vi "CtrlTreeUpdateModifiedState.vi"(7 "Selection":string, 10 "ControlTree in":refnum<vi>, 11 "SavedSettings in":refnum<vi>) -> (1 "Boolean":bool)   [LabVIEW 2020]
panel:
  in  "error in (no error)":errorcluster
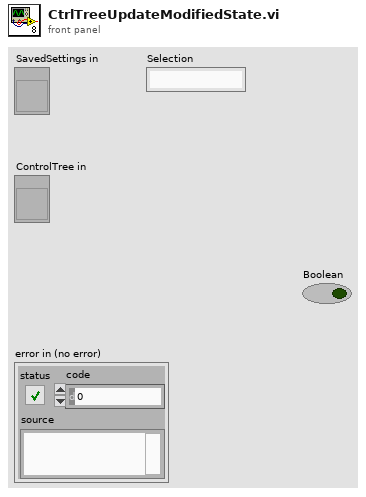
[diagram p1: front panel]
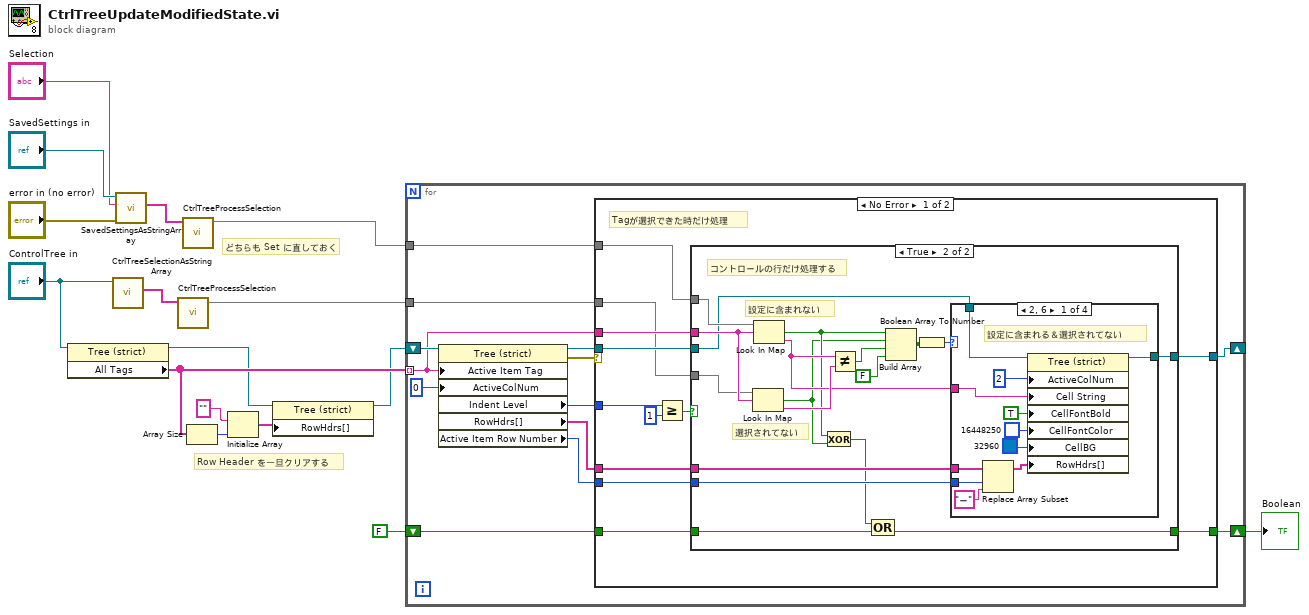
[diagram p0: block diagram]
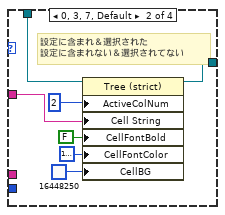
[diagram p3: hidden frame]
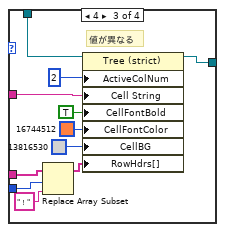
[diagram p4: hidden frame]
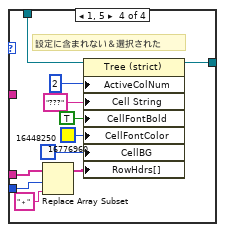
[diagram p5: hidden frame]
diagram:
  # "Row Header を一旦クリアする"
  # "どちらも Set に直しておく"
  n1 = property class="Tree (strict)"(reference="ControlTree in") -> (reference out=w6:refnum<vi>, "All Tags"=w9:string[])  [unwired: 1 in, 1 out]
  n2 = call "CtrlTreeSelectionAsStringArray.vi"("TreeControl in"="ControlTree in") -> ("Selection"=w15:string[])  [unwired: 8 in, 2 out]
  n3 = call "SavedSettingsAsStringArray.vi"("error in (no error)"="error in (no error)", "Tag"="Selection", "SavedSettings in"="SavedSettings in") -> ("Selection"=w2:string[])  [unwired: 4 in, 4 out]
  n4 = call "CtrlTreeProcessSelection.vi"("Selection"=w15) -> ("Map"=w4:map{string, string})  [unwired: 10 in]
  n5 = call "CtrlTreeProcessSelection.vi"("Selection"=w2) -> ("Map"=w3:map{string, string})  [unwired: 10 in]
  n6 = Array Size(array=w9) -> (size(s)=w10:i32)
  n7 = Initialize Array("", w10) -> (w7:string[])
  n8 = property class="Tree (strict)"(reference=w6, "RowHdrs[]"=w7) -> (reference out=w5:refnum<vi>)  [unwired: 1 in, 1 out]
  n9 = for {
    tunnel: w9 -> [w26] mode=indexing
    tunnel: w4 -> [w23]
    tunnel: w3 -> [w24]
    shift-right: [w21] -> w12
    shift-left: FALSE -> [w20]
    shift-right: [w17] -> _
    shift-left: w5 -> [w29]
    n10 = property class="Tree (strict)"(reference=w29, "Active Item Tag"=w26, "ActiveColNum"=0 ("Active Cell:Active Column Number")) -> (reference out=w27:refnum<vi>, error out=w22:errorcluster, "Indent Level"=w25:i32, "RowHdrs[]"=w19:string[], "Active Item Row Number"=w18:i32)  [unwired: 1 in]
    n11 = case shown="No Error" w22 {
      tunnel: w27 -> [w41 w102]
      tunnel: w26 -> [w40 _]
      tunnel: w25 -> [w39 _]
      tunnel: w24 -> [w38 _]
      tunnel: w23 -> [w37 _]
      tunnel: [w36 w103] -> w21
      tunnel: w20 -> [w35 w103]
      tunnel: w19 -> [w34 _]
      tunnel: w18 -> [w33 _]
      tunnel: [w32 w102] -> w17
      frame No Error {
        # "Tagが選択できた時だけ処理"
        n12 = Greater Or Equal?(x=w39, y=1) -> (x >= y?=w30:bool)
        n13 = case shown="True" w30 {
          tunnel: w40 -> [_ w60]
          tunnel: w38 -> [_ w59]
          tunnel: w37 -> [_ w58]
          tunnel: w41 -> [w42 w54]
          tunnel: [w43 w51] -> w36
          tunnel: w35 -> [w43 w52]
          tunnel: w34 -> [_ w50]
          tunnel: w33 -> [_ w49]
          tunnel: [w42 w44] -> w32
          frame False {
          }
          frame True {
            # "コントロールの行だけ処理する"
            # "設定に含まれない"
            # "選択されてない"
            n14 = Look In Map(map=w58, key=w60) -> (key not found?=w46:bool, value=w61:string)  [unwired: 1 in]
            n15 = Look In Map(map=w59, key=w60) -> (key not found?=w47:bool, value=w53:string)  [unwired: 1 in]
            n16 = Exclusive Or(1:w46, 2:w47) -> (0:w45:bool)
            n17 = Not Equal?(x=w53, y=w61) -> (x != y?=w57:bool)
            n18 = Compound Arithmetic op=OR(w45, w52) -> (w51:bool)
            n19 = Build Array(w47, w46, w57, FALSE ("element")) -> (w56:bool[])
            n20 = Boolean Array To Number(Boolean array=w56) -> (number=w55:u32)
            n21 = case shown="2, 6" w55 {
              tunnel: w54 -> [w70 w76 w86 w97]
              tunnel: w53 -> [w69 w74 w85 _]
              tunnel: w50 -> [w65 _ w82 w95]
              tunnel: w49 -> [w64 _ w81 w94]
              tunnel: [w62 w73 w80 w91] -> w44
              frame 2, 6 {
                # "設定に含まれる＆選択されてない"
                n22 = Replace Array Subset(array=w65, new element="ー" ("new element/subarray"), index=w64) -> (w63:string[])
                n23 = property class="Tree (strict)"(reference=w70, "ActiveColNum"=2 ("Active Cell:Active Column Number"), "Cell String"=w69, "CellFontBold"=TRUE ("Active Cell:Cell Font:Bold"), "CellFontColor"=u32 16448250 ("Active Cell:Cell Font:Color"), "CellBG"=u32 32960 ("Active Cell:Cell Font:Color"), "RowHdrs[]"=w63) -> (reference out=w62:refnum<vi>)  [unwired: 1 in, 1 out]
              }
              frame 0, 3, 7, Default {
                # "設定に含まれ＆選択された\n設定に含まれない＆選択されてない"
                n24 = property class="Tree (strict)"(reference=w76, "ActiveColNum"=2 ("Active Cell:Active Column Number"), "Cell String"=w74, "CellFontBold"=FALSE ("Active Cell:Cell Font:Bold"), "CellFontColor"=u32 16777228 ("Active Cell:Cell Font:Color"), "CellBG"=u32 16448250 ("Active Cell:Cell Font:Color")) -> (reference out=w73:refnum<vi>)  [unwired: 1 in, 1 out]
              }
              frame 4 {
                # "値が異なる"
                n25 = Replace Array Subset(array=w82, new element="！" ("new element/subarray"), index=w81) -> (w83:string[])
                n26 = property class="Tree (strict)"(reference=w86, "ActiveColNum"=2 ("Active Cell:Active Column Number"), "Cell String"=w85, "CellFontBold"=TRUE ("Active Cell:Cell Font:Bold"), "CellFontColor"=u32 16744512 ("Active Cell:Cell Font:Color"), "CellBG"=u32 13816530 ("Active Cell:Cell Font:Color"), "RowHdrs[]"=w83) -> (reference out=w80:refnum<vi>)  [unwired: 1 in, 1 out]
              }
              frame 1, 5 {
                # "設定に含まれない＆選択された"
                n27 = Replace Array Subset(array=w95, new element="＋" ("new element/subarray"), index=w94) -> (w93:string[])
                n28 = property class="Tree (strict)"(reference=w97, "ActiveColNum"=2 ("Active Cell:Active Column Number"), "Cell String"="???" ("Active Cell:String"), "CellFontBold"=TRUE ("Active Cell:Cell Font:Bold"), "CellFontColor"=u32 16776960 ("Active Cell:Cell Font:Color"), "CellBG"=u32 16448250 ("Active Cell:Cell Font:Color"), "RowHdrs[]"=w93) -> (reference out=w91:refnum<vi>)  [unwired: 1 in, 1 out]
              }
            }
          }
        }
      }
      frame Error {
      }
    }
  }
  "Boolean" <- w12
